vi "dsdll_vi_tree.vi"   [LabVIEW 2020, in "dsdll.lvlib"]
doc: "DirectSound interface VI tree."
uses:
  dsdll.lvlib
  dsdll_output_write_auto_float32.vi
  dsdll_capture_wave_byte_array.vi
panel:
  # "DS DLL\nVI Tree"
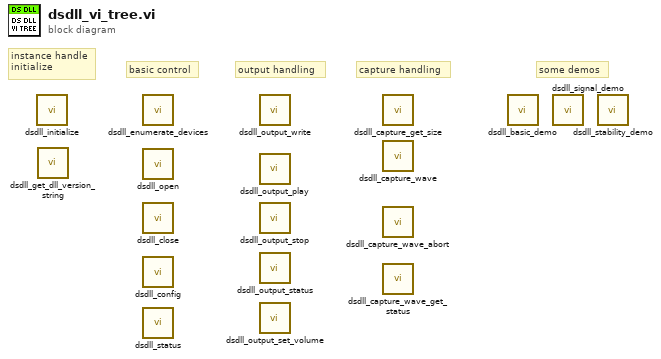
[diagram p0: block diagram]
diagram:
  # "some demos"
  # "capture handling"
  # "output handling"
  # "basic control"
  # "instance handle\ninitialize"
  n1 = call "dsdll_initialize.vi"() -> ()  [unwired: 10 in, 2 out]
  n2 = call "dsdll_get_dll_version_string.vi"() -> ()  [unwired: 9 in, 3 out]
  n3 = call "dsdll_enumerate_devices.vi"() -> ()  [unwired: 8 in, 4 out]
  n4 = call "dsdll_open.vi"() -> ()  [unwired: 10 in, 2 out]
  n5 = call "dsdll_close.vi"() -> ()  [unwired: 10 in, 2 out]
  n6 = call "dsdll_config.vi"() -> ()  [unwired: 10 in, 2 out]
  n7 = call "dsdll_status.vi"() -> ()  [unwired: 6 in, 6 out]
  n8 = call-poly "dsdll_output_write.vi"() -> ()  [unwired: 10 in, 2 out]
  n9 = call "dsdll_output_play.vi"() -> ()  [unwired: 10 in, 2 out]
  n10 = call "dsdll_output_stop.vi"() -> ()  [unwired: 10 in, 2 out]
  n11 = call "dsdll_output_status.vi"() -> ()  [unwired: 5 in, 7 out]
  n12 = call "dsdll_output_set_volume.vi"() -> ()  [unwired: 10 in, 2 out]
  n13 = call "dsdll_capture_get_size.vi"() -> ()  [unwired: 6 in, 6 out]
  n14 = call-poly "dsdll_capture_wave.vi"() -> ()  [unwired: 4 in, 8 out]
  n15 = call "dsdll_capture_wave_abort.vi"() -> ()  [unwired: 9 in, 3 out]
  n16 = call "dsdll_capture_wave_get_status.vi"() -> ()  [unwired: 6 in, 6 out]
  n17 = call "dsdll_basic_demo.vi"() -> ()  [unwired: 12 in]
  n18 = call "dsdll_signal_demo.vi"() -> ()  [unwired: 12 in]
  n19 = call "dsdll_stability_demo.vi"() -> ()  [unwired: 12 in]
